vi "限幅器（U16）.vi"(3 "下限":u16, 4 "X_in":u16, 5 "上限":u16) -> (1 "X_Out":u16)   [LabVIEW 2012]
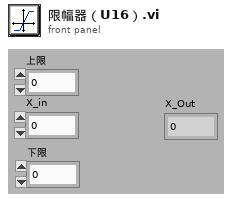
[diagram p1: front panel]
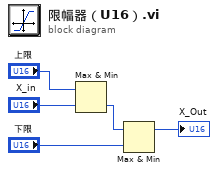
[diagram p0: block diagram]
diagram:
  n1 = Max & Min(x="上限", y="X_in") -> (min(x,y)=w3:u16)  [unwired: 1 out]
  n2 = Max & Min(x=w3, y="下限") -> (max(x,y)=→"X_Out":u16)  [unwired: 1 out]
